vi "Configure ISIM Security.vi"(0 "VISA resource name":refnum<visa-resource-name>, 1 "Authentication Management Field (\"\")":string, 2 "Operator Code Value (\"\")":string, 5 "SIM Profile Name (\"\")":string, 7 "Authentication Algorithm (Milenage)":i32(ring) items=["Milenage", "XOR"], 9 "Secret Key (\"\")":string, 11 "error in (no error)":errorcluster, 12 "Operator Code Type (Ciphered)":i32(ring) items=["Ciphered", "Plain"], 13 "Sequence Number Incrementation (Off)":bool) -> (4 "VISA resource name out":refnum<visa-resource-name>, 15 "error out":errorcluster)   [LabVIEW 2020, in "Rohde&Schwarz CMXP Base.lvlib"]
doc: "Configures ISIM Security Settings\n\nAttributes:\nRSCMXPBASE_ATTR_ISIM_AUTHENTICATION_ALGORITHM\nRSCMXPBASE_ATTR_ISIM_SECRET_KEY\nRSCMXPBASE_ATTR_ISIM_AUTHENTICATION_MANAGEMENT_FIELD\nRSCMXPBASE_ATTR_ISIM_OPERATOR_CODE\nRSCMXPBASE_ATTR_ISIM_INCREMENTS_SEQUENCE_NUMBER_ENABLED\n\nRemote-control commands:\n[CONFigure:]SIMProfile:ISIM:SECurity:AUTHentic\n[CONFigure:]SIMProfile:ISIM:SECurity:SKEY\n[CONFigure:]SIMProfile:ISIM:SECurity:AMField\n[CONFigure:]SIMProfile:ISIM:SECurity:OCODe\n[CONFigure:]SIMProfile:ISIM:SECurity:SNINcrement"
uses:
  <instrlib>/Rohde&Schwarz CMXP Base/Rohde&Schwarz CMXP Base.lvlib
  <instrlib>/Rohde&Schwarz CMXP Base/Private/rsidr_core.llb/rsidr_core.lvlib
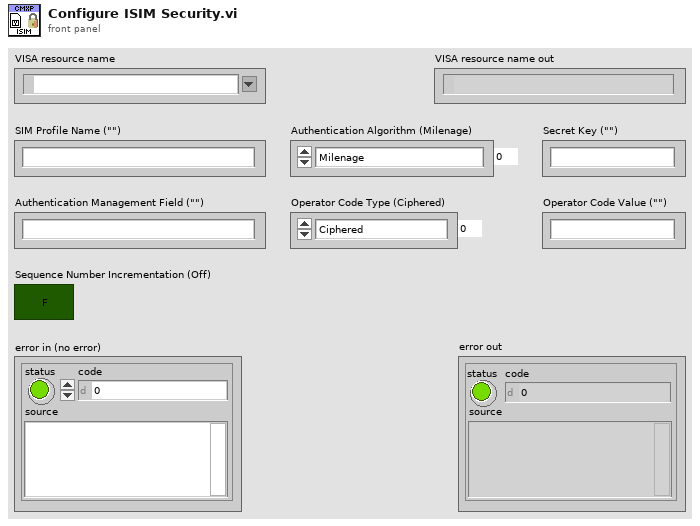
[diagram p1: front panel]
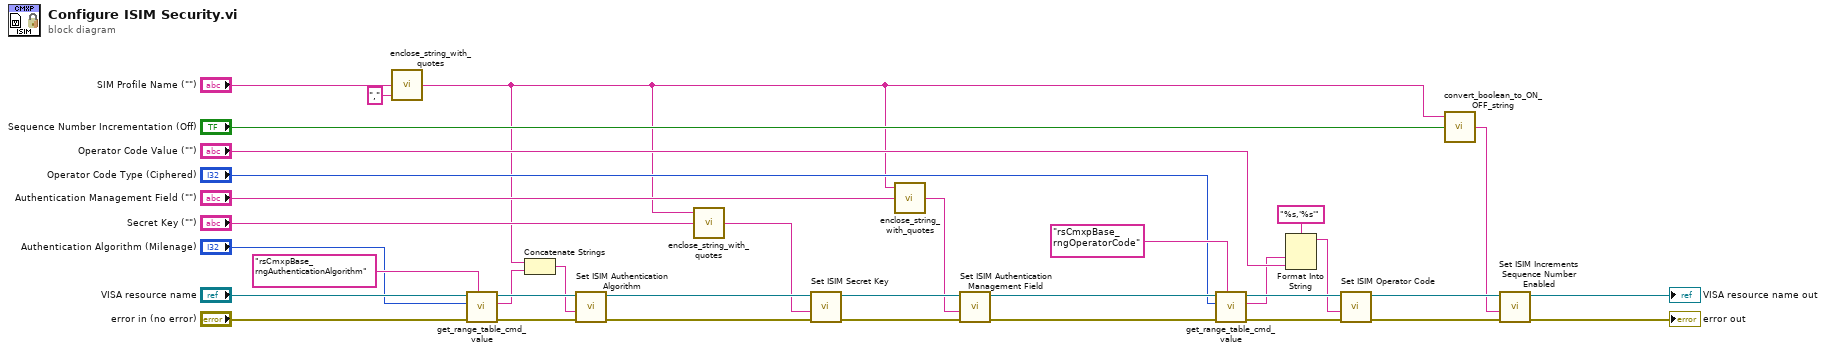
[diagram p0: block diagram]
diagram:
  n1 = call <instrlib>:"enclose_string_with_quotes.vi"("String after"=",", "String to enclose"="SIM Profile Name (\"\")") -> ("String out"=w2:string)  [unwired: 3 in]
  n2 = call <instrlib>:"get_range_table_cmd_value.vi"("Range Table ID in"="rsCmxpBase_rngAuthenticationAlgorithm", "error in"="error in (no error)", "Input Int32 value"="Authentication Algorithm (Milenage)", "VISA resource name"="VISA resource name") -> ("error out"=w35:errorcluster, "Cmd value out"=w8:string, "VISA resource name out"=w34:refnum<visa-resource-name>)  [unwired: 5 in]
  n3 = Concatenate Strings(w2, w8) -> (w11:string)
  n4 = call "Set ISIM Authentication Algorithm"("error in (no error)"=w35, "ISIM Authentication Algorithm ()"=w11, "instrument handle"=w34) -> ("error out"=w32:errorcluster, "instrument handle out"=w31:refnum<visa-resource-name>)  [unwired: 7 in]
  n5 = call <instrlib>:"enclose_string_with_quotes.vi"("String to enclose"="Secret Key (\"\")", "String before"=w2) -> ("String out"=w4:string)  [unwired: 3 in]
  n6 = call "Set ISIM Secret Key"("error in (no error)"=w32, "ISIM Secret Key ()"=w4, "instrument handle"=w31) -> ("error out"=w30:errorcluster, "instrument handle out"=w29:refnum<visa-resource-name>)  [unwired: 7 in]
  n7 = call <instrlib>:"enclose_string_with_quotes.vi"("String to enclose"="Authentication Management Field (\"\")", "String before"=w2) -> ("String out"=w1:string)  [unwired: 3 in]
  n8 = call "Set ISIM Authentication Management Field"("error in (no error)"=w30, "ISIM Authentication Management Field ()"=w1, "instrument handle"=w29) -> ("error out"=w26:errorcluster, "instrument handle out"=w25:refnum<visa-resource-name>)  [unwired: 7 in]
  n9 = call <instrlib>:"get_range_table_cmd_value.vi"("Range Table ID in"="rsCmxpBase_rngOperatorCode", "error in"=w26, "Input Int32 value"="Operator Code Type (Ciphered)", "VISA resource name"=w25) -> ("error out"=w24:errorcluster, "Cmd value out"=w10:string, "VISA resource name out"=w23:refnum<visa-resource-name>)  [unwired: 5 in]
  n10 = Format Into String(format string="%s,'%s'", w10, "Operator Code Value (\"\")") -> (resulting string=w12:string)  [unwired: 2 in, 1 out]
  n11 = call "Set ISIM Operator Code"("error in (no error)"=w24, "ISIM Operator Code ()"=w12, "instrument handle"=w23) -> ("error out"=w28:errorcluster, "instrument handle out"=w27:refnum<visa-resource-name>)  [unwired: 7 in]
  n12 = call <instrlib>:"convert_boolean_to_ON_OFF_string.vi"("boolean value in"="Sequence Number Incrementation (Off)", "String to add before (\"\")"=w2) -> ("string value out"=w13:string)  [unwired: 3 in]
  n13 = call "Set ISIM Increments Sequence Number Enabled"("error in (no error)"=w28, "ISIM Increments Sequence Number Enabled ()"=w13, "instrument handle"=w27) -> ("error out"=→"error out":errorcluster, "instrument handle out"=→"VISA resource name out":refnum<visa-resource-name>)  [unwired: 7 in]
